vi "Test Program Write Tag.vi"(8 "error in (no error)":errorcluster, 10 "data":waveform(dbl)[](array[waveform]), 11 "Data Cluster":T1) -> (0 "error out":errorcluster, 1 "Data Cluster 3":T1, 2 "DAQ value":dbl format="%0.2f", 3 "Y":dbl[](array[numeric]))   [LabVIEW 2018, in "DAQ.lvlib"]
uses:
  DAQ.lvlib
  <vilib>/Analysis/baseanly.llb/Mean (DBL).vi
  <vilib>/Analysis/NI_AALBase.lvlib
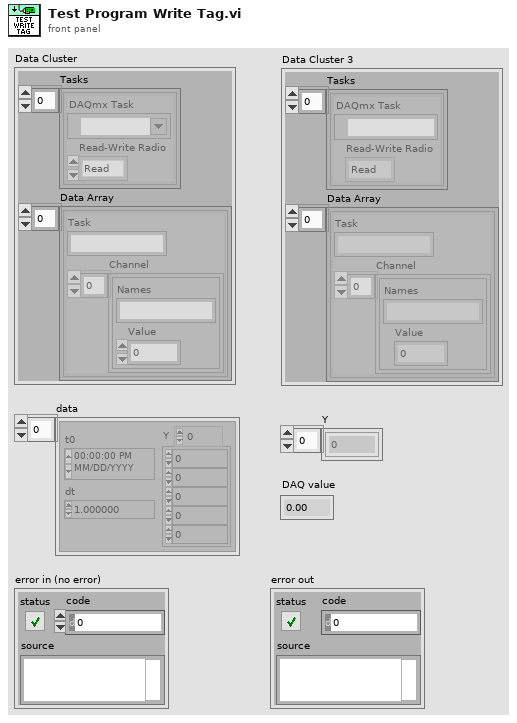
[diagram p1: front panel]
types:
  T1 = cluster{"Tasks":cluster{"DAQmx Task":refnum<k21>, "Read-Write Radio":enum32{"Read", "Write"}}[], "Data Array":cluster{"Task":string, "Channel":cluster{"Names":string, "Value":dbl}[]}[]}
  T2 = cluster{"Task":string, "Channel":cluster{"Names":string, "Value":dbl}[]}[]
  T3 = cluster{"Task":string, "Channel":cluster{"Names":string, "Value":dbl}[]}
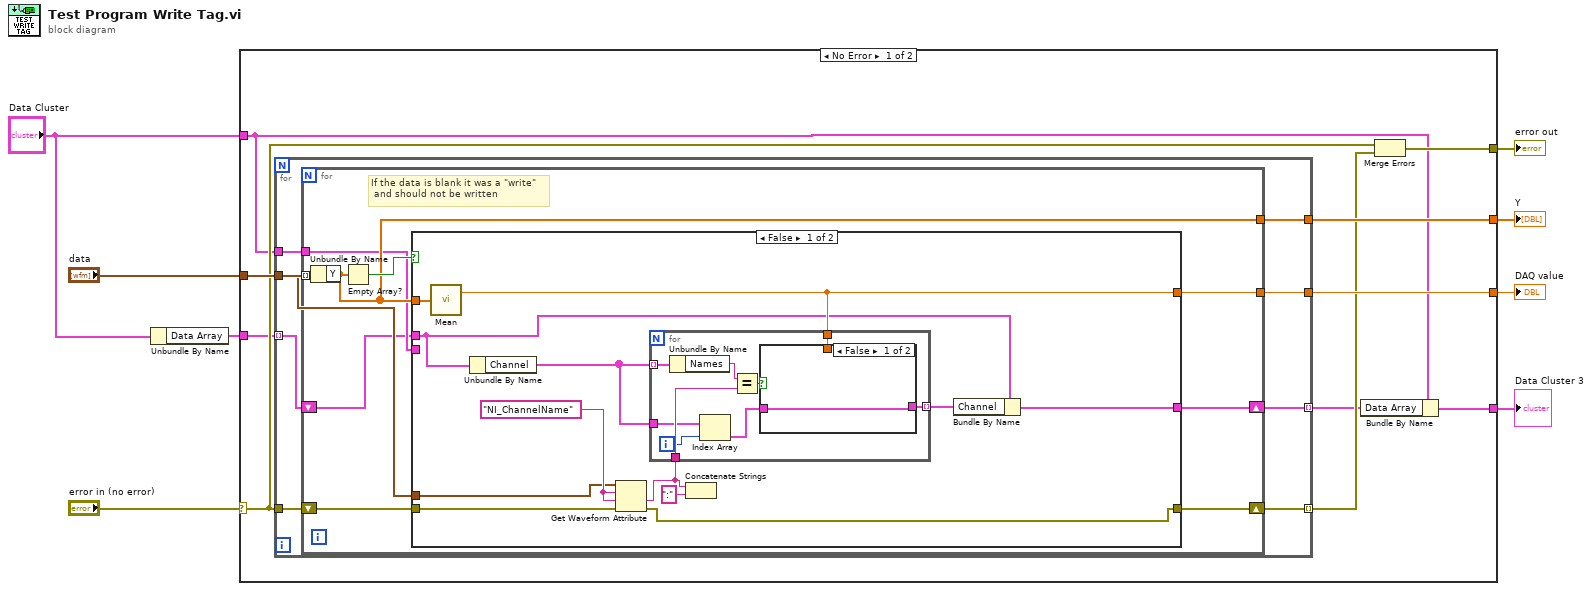
[diagram p0: block diagram]
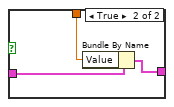
[diagram p2: hidden frame]
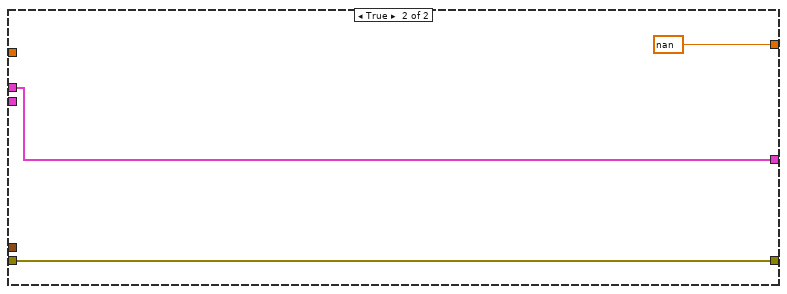
[diagram p3: hidden frame]
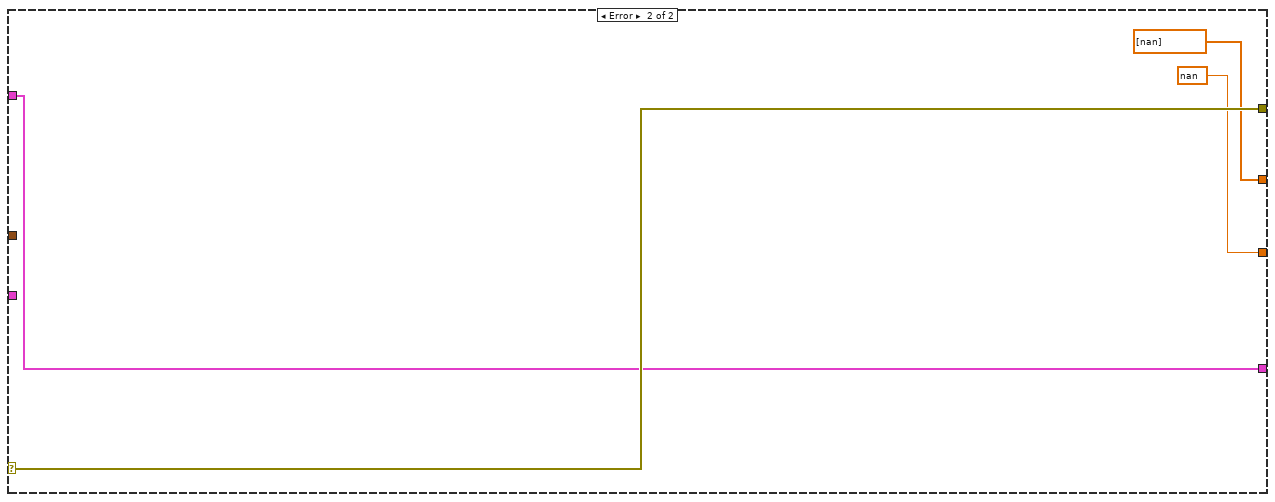
[diagram p4: hidden frame]
diagram:
  n1 = Unbundle By Name("Data Cluster") -> ("Data Array"=w6:T2)
  n2 = case shown="No Error" "error in (no error)" {
    selector: "error in (no error)" -> [w13 w67]
    tunnel: [w14 w67] -> w1
    tunnel: "data" -> [w18 _]
    tunnel: [w17 nan ("mean")] -> w3
    tunnel: [w16 dbl[] [nan] ("Y")] -> w4
    tunnel: w6 -> [w12 _]
    tunnel: "Data Cluster" -> [w11 w64]
    tunnel: [w9 w64] -> w8
    frame No Error {
      n3 = for {
        tunnel: w18 -> [w26]
        tunnel: w13 -> [w25]
        tunnel: [w24] -> w15 mode=indexing
        tunnel: [w23] -> w17
        tunnel: [w22] -> w16
        tunnel: w12 -> [w19] mode=indexing
        tunnel: w11 -> [w21]
        tunnel: [w20] -> w10 mode=indexing
        n4 = for {
          tunnel: w26 -> [w35] mode=indexing
          tunnel: [w31] -> w23
          tunnel: [w30] -> w22
          tunnel: w21 -> [w29]
          shift-right: [w32] -> w24
          shift-left: w25 -> [w33]
          shift-right: [w28] -> w20
          shift-left: w19 -> [w27]
          # "If the data is blank it was a \"write\"\n and should not be written"
          n5 = Unbundle By Name(w35) -> ("Y"=w30:dbl[])
          n6 = Empty Array?(array=w30) -> (empty?=w34:bool)
          n7 = case shown="False" w34 {
            tunnel: w35 -> [w46 _]
            tunnel: w30 -> [w44 _]
            tunnel: w33 -> [w45 w62]
            tunnel: [w43 w62] -> w32
            tunnel: [w40 nan ("mean")] -> w31
            tunnel: w27 -> [w39 w61]
            tunnel: w29 -> [_ _]
            tunnel: [w37 w61] -> w28
            frame False {
              w47 = "NI_ChannelName" ("name")
              n8 = call-poly <vilib>:"Mean.vi"("X"=w44) -> ("mean"=w40:dbl)  [unwired: 1 out]
              n9 = Unbundle By Name(w39) -> ("Channel"=w36:cluster{"Names":string, "Value":dbl}[])
              n10 = Get Waveform Attribute(4:w45, 5:w47, 6:w47, 7:w46) -> (0:w43:errorcluster, 1:w41:string)  [unwired: 2 out]
              n11 = for {
                tunnel: w41 -> [w56]
                tunnel: w36 -> [w53] mode=indexing
                tunnel: w40 -> [w52]
                tunnel: [w51] -> w38 mode=indexing
                tunnel: w36 -> [w49]
                i -> [w50]
                n12 = Unbundle By Name(w53) -> ("Names"=w54:string)
                n13 = Index Array(array=w49, index=w50) -> (element=w48:cluster{"Names":string, "Value":dbl})
                n14 = Equal?(x=w54, y=w56) -> (x = y?=w55:bool)
                n15 = case shown="False" w55 {
                  tunnel: w48 -> [w57 w60]
                  tunnel: w52 -> [_ w59]
                  tunnel: [w57 w58] -> w51
                  frame False {
                  }
                  frame True {
                    n16 = Bundle By Name(cluster=w60, "Value"=w59) -> (w58:cluster{"Names":string, "Value":dbl})
                  }
                }
              }
              n17 = Concatenate Strings(w41, ":" ("string")) -> ()  [unwired: 1 out]
              n18 = Bundle By Name(cluster=w39, "Channel"=w38) -> (w37:T3)
            }
            frame True {
            }
          }
        }
      }
      n19 = Bundle By Name(cluster=w11, "Data Array"=w10) -> (w9:T1)
      n20 = Merge Errors(w13, w15) -> (w14:errorcluster)
    }
    frame Error {
    }
  }
  "error out" <- w1
  "DAQ value" <- w3
  "Y" <- w4
  "Data Cluster 3" <- w8
